vi "Global_PUMP.vi"() -> ()   [LabVIEW 2015]
panel:
  out "PUMP ready":bool
  out "PUMP done":bool
  out "PUMP start":bool
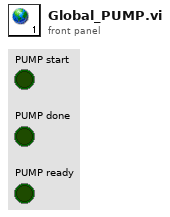
[diagram p1: front panel]
diagram:
